vi "LeddarClose.vi"(10 "Event Callback":refnum<k27>, 11 "DeviceControl":refnum<k24>) -> ()   [LabVIEW 2012]
uses:
  C:/Program Files/LeddarTech/xtec/LeddarNET2.dll
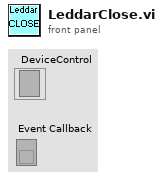
[diagram p1: front panel]
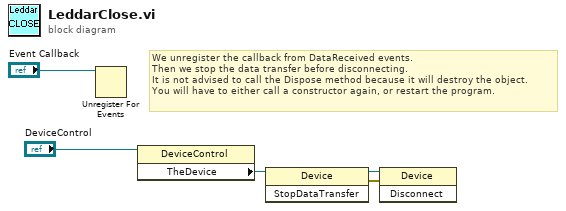
[diagram p0: block diagram]
diagram:
  # "We unregister the callback from DataReceived events.\nThen we stop the data transfer before disconnecting.\nIt is not advised to call the Dispose method because it will destroy the object.\nYou will have to either call a constructor again, or restart the program."
  n1 = Unregister For Events(event registration refnum="Event Callback") -> ()  [unwired: 1 in, 1 out]
  n2 = property class="DeviceControl"(reference="DeviceControl") -> ("TheDevice"=w5:refnum<k24>)  [unwired: 1 in, 2 out]
  n3 = invoke class="Device" method="StopDataTransfer"(reference=w5) -> (reference out=w3:refnum<k24>, error out=w1:errorcluster)  [unwired: 2 in, 1 out]
  n4 = invoke class="Device" method="Disconnect"(reference=w3, error in=w1) -> ()  [unwired: 1 in, 3 out]
